vi "Update UI.vi"(11 "Mediator in":refnum<class "Mediator.lvclass">) -> (3 "Mediator out":refnum<class "Mediator.lvclass">)   [LabVIEW 2015, in "Mediator.lvlib" / "Mediator.lvclass"]
uses:
  Mediator.lvclass
  Mediator.lvclass/Mediator.ctl
  TopicLookupTable/TopicLookupTable.lvclass
panel:
  out "error out":errorcluster
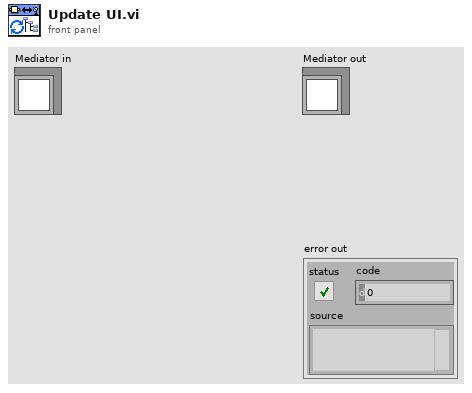
[diagram p1: front panel]
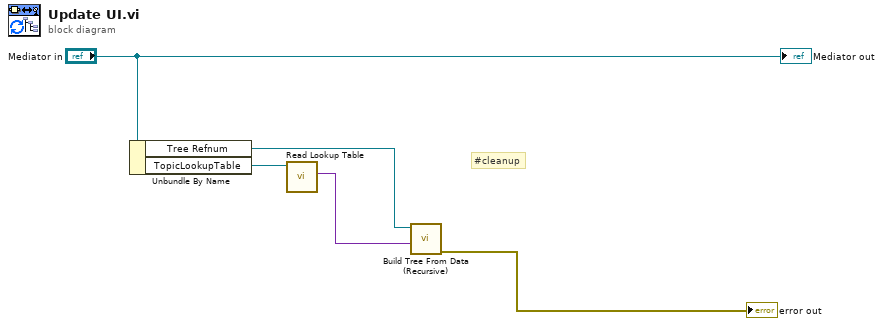
[diagram p0: block diagram]
diagram:
  # "#cleanup"
  n1 = Unbundle By Name("Mediator in") -> ("Tree Refnum"=w2:refnum<vi>, "TopicLookupTable"=w4:refnum<class "TopicLookupTable.lvclass">)
  n2 = call "Read Lookup Table.vi"("TopicLookupTable in"=w4) -> ("Topic Table"=w3:variant)  [unwired: 10 in]
  n3 = call "Build Tree From Data (Recursive).vi"("Variant"=w3, "TreeControl Ref"=w2) -> ("error out"=→"error out":errorcluster)  [unwired: 7 in, 2 out]
  "Mediator out" <- "Mediator in"
